vi "Read (Calculation).vi"(8 "error in (no error)":errorcluster, 9 "Maximum Time (10000 ms)":u32=10000, 11 "VISA resource name":refnum<visa-resource-name>) -> (0 "error out":errorcluster, 1 "Minimum":dbl format="%#.10g", 2 "Standard Deviation":dbl format="%#.10g", 3 "VISA resource name out":refnum<visa-resource-name>, 4 "Maximum":dbl format="%#.10g", 5 "Mean":dbl format="%#_10g")   [LabVIEW 2020, in "Counter.lvlib" / "PICOTEST U62XXA series.lvlib"]
doc: "Reads and returns all four Statistics generated from a series of measurements.\n\n<B>Note:</B>\n\nIf no valid result exists, Not a Number 9.91E37 is returned."
uses:
  PICOTEST U62XXA series.lvlib
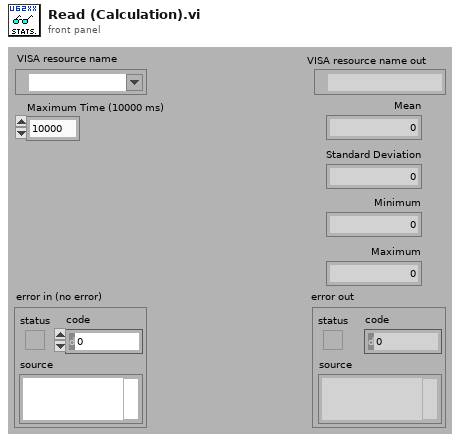
[diagram p1: front panel]
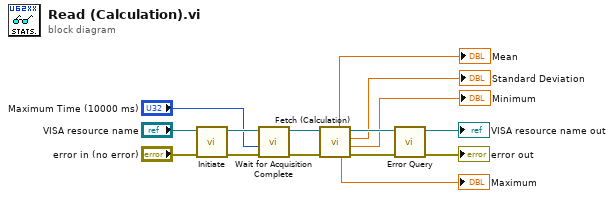
[diagram p0: block diagram]
diagram:
  n1 = call "Initiate.vi"("error in (no error)"="error in (no error)", "VISA resource name"="VISA resource name") -> ("error out"=w8:errorcluster, "VISA resource name out"=w9:refnum<visa-resource-name>)  [unwired: 8 in]
  n2 = call "Wait for Acquisition Complete.vi"("error in (no error)"=w8, "Maximum Time (10000 ms)"="Maximum Time (10000 ms)", "VISA resource name"=w9) -> ("error out"=w2:errorcluster, "VISA resource name out"=w3:refnum<visa-resource-name>)  [unwired: 7 in]
  n3 = call "Fetch (Calculation).vi"("error in (no error)"=w2, "VISA resource name"=w3) -> ("error out"=w11:errorcluster, "Minimum"=→"Minimum":dbl, "Standard Deviation"=→"Standard Deviation":dbl, "VISA resource name out"=w14:refnum<visa-resource-name>, "Maximum"=→"Maximum":dbl, "Mean"=→"Mean":dbl)  [unwired: 4 in]
  n4 = call "Error Query.vi"("error in (no error)"=w11, "VISA resource name"=w14) -> ("error out"=→"error out":errorcluster, "VISA resource name out"=→"VISA resource name out":refnum<visa-resource-name>)  [unwired: 6 in, 2 out]
